vi "FXP_AFMss_MPC_singleAxis.vi"() -> ()   [LabVIEW 2017]
uses:
  <vilib>/eio/EIONode/EIONode.xnode
  <vilib>/rvi/eio/common/nirviEmuTemplateMethod_errors.vi
  <vilib>/rvi/DataTransferAndStorage/Container/XNode/niFpgaContainer.xnode
  <vilib>/eio/EIOGrowableMethodNode/genericMethod/EIOGrowableMethodNode.xnode
  <vilib>/rvi/eio/nirviErrorMerge/nirviErrorMerge.xnode
  <vilib>/rvi/eio/nirviEIOMethodImplementation/nirviEIOMethodImplementation.xnode
  <vilib>/rvi/eio/common/nirviEmuClasses.ctl
  <vilib>/rvi/FXPMathLib/FxpSub/XNode/nifxpmath_Sub.xnode
  <vilib>/Platform/TimedLoop/XDataNode/XDataNode.xnode
  <vilib>/Platform/TimedLoop/XDataNode/nitl_modes.ctl
  <vilib>/Platform/TimedLoop/XDataNode/XDNodeRunTimeDep.lvlib
  <vilib>/Platform/TimedLoop/XDataNode/wakeup.ctl
  <vilib>/Platform/TimedLoop/XDataNode/timing_clust.ctl
  <vilib>/rvi/FXPMathLib/sim/FxpSim.dll
  <vilib>/rvi/interface/RandomDataEmulation/nirviRandomDataFpgaReadWriteTemplate.vi
  fpga_fp_interface_lib/fpga_interface_types/boolean_indicators.ctl
  <vilib>/rvi/Memory/Memory_Emulation/nirvimemoryFastEmulation.vi
  <vilib>/rvi/Memory/Memory_Emulation/nirvimemoryEmulation.vi
  typeDefs/FXPControlParams_distEst.ctl
  fgm_pipiline/quadProgParams_pipe.ctl
panel:
  in  "ControlParams_distEst":T1={"umax"=3.0, "NS"=0, "ref_f_VEC"=[0.0, 0.0], "du_max"=0.0}
  in  "QP_params":T2={"maxIter"=0, "nuN"=24, "Ns_mpc"=0, "-beta"=-0.9987945556640625, "beta+1"=1.9987945556640625}
  out "Matrix FIFO \nTimeOut":bool
  out "u_k out":fxp<+/-,32,5>
  out "boolean  indicators":T3
  out "x-x(0)":fxp<+/-,18,5>
  out "y-axis fast":fxp<+/-,16,5>
  out "x(0)":fxp<+/-,16,5>
  out "LoopTicks2":u32
  out "Error Out":errorcluster
  out "x-axis fast":fxp<+/-,16,5>
  out "AI Timed Out":bool
  out "Stopped":bool
  in  "Settle Ticks":i16=1000
  in  "iters":i16=1
  in  "ymax":fxp<+/-,32,16>=4.0
  in  "TsTicks":i16
  out "Loop Ticks (benchmark)":i16
  out "NS":u8=2
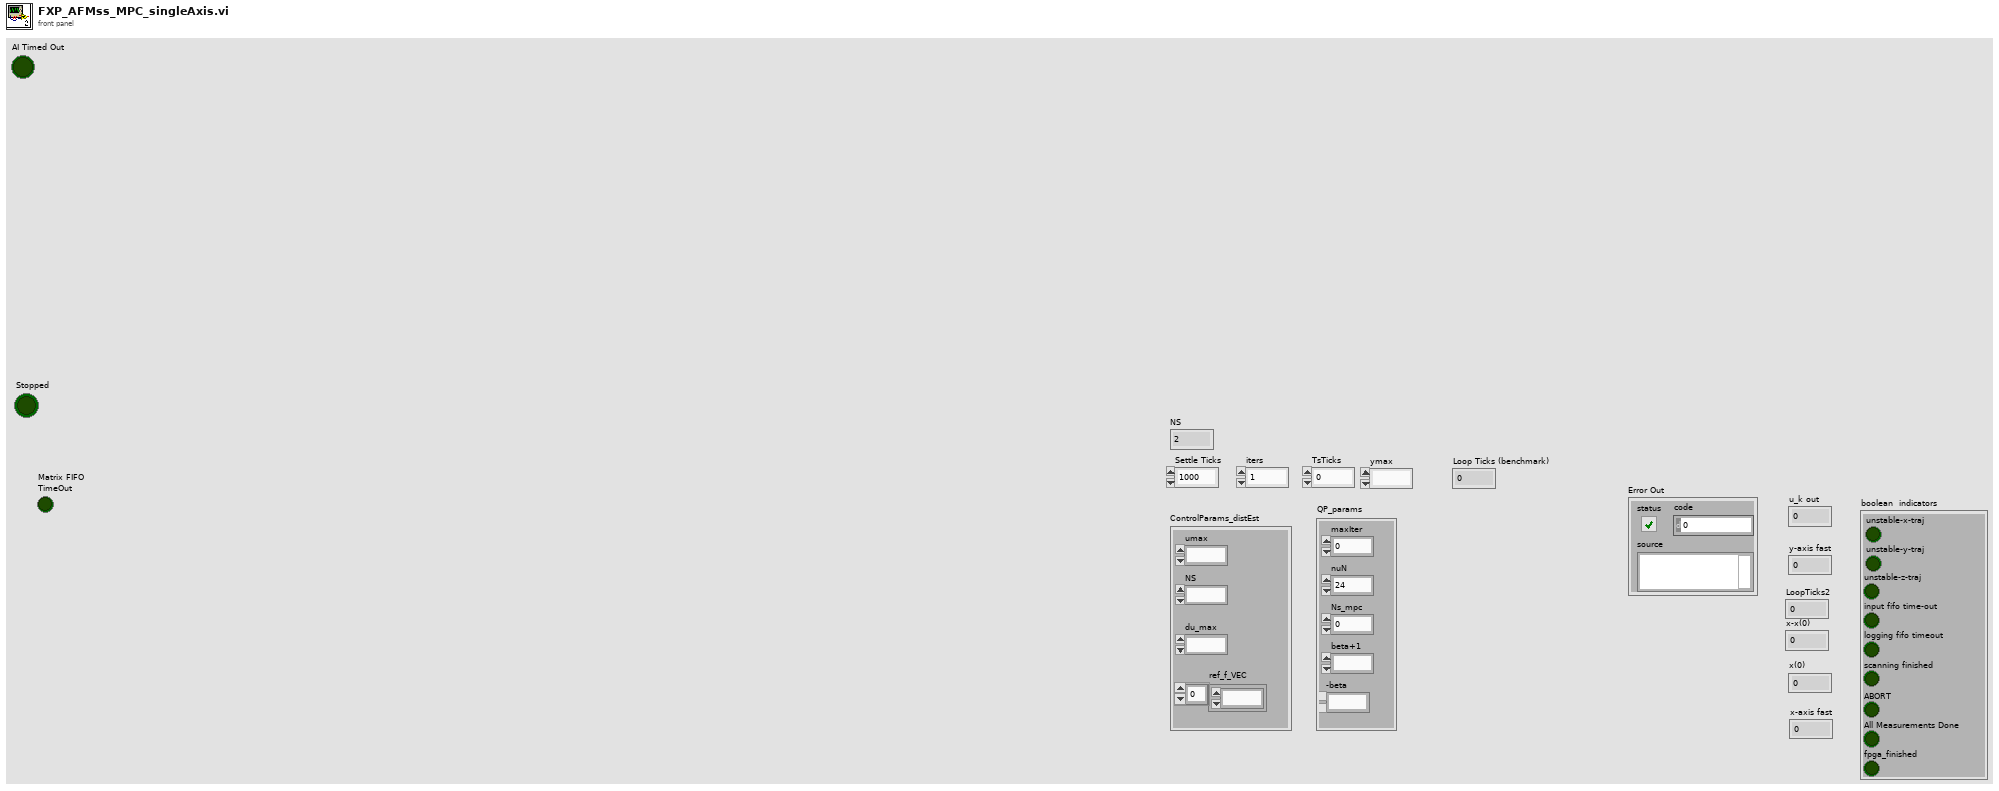
[diagram p1: front panel]
types:
  T1 = typedef "FXPControlParams_distEst.ctl" = cluster{"umax":fxp<+/-,18,5>, "NS":u8, "ref_f_VEC":fxp<+/-,32,5>[], "du_max":fxp<+/-,18,5>}
  T2 = typedef "quadProgParams_pipe.ctl" = cluster{"maxIter":u16, "nuN":u16, "Ns_mpc":u16, "-beta":fxp<+/-,18,2>, "beta+1":fxp<+/-,18,2>}
  T3 = typedef "boolean_indicators.ctl" = cluster{"unstable-z-traj":bool, "input fifo time-out":bool, "logging fifo timeout":bool, "scanning finished":bool, "unstable-x-traj":bool, "unstable-y-traj":bool, "ABORT":bool, "All Measurements Done":bool, "fpga_finished":bool}
  T4 = typedef "nirviEmuClasses.ctl" = enum16{"IO Read", "IO Write", "Method", "Property Read", "Property Write"}
  T5 = typedef "XDNodeRunTimeDep.lvlib/timing_clust.ctl" = cluster{"Expected End [f-1]":u64, "Actual End [f-1]":u64, "Finished Late? [f-1]":bool, "Expected End [i-1]":u64, "Actual End [i-1]":u64, "Finished Late? [i-1]":bool, "Expected Start [i]":u64, "Actual Start [i]":u64, "Expected Start [f]":u64, "Actual Start [f]":u64, "Source Name":string, "Structure Name":string, "Period":i64, "Deadline":i64, "Offset":i64, "Start":i64, "Priority":i32, "Timeout":i32, "Mode":T6, "Wakeup Reason":T7, "Error":errorcluster, "Source Type":string, "Secondary Source Type":string, "Global End Time":u64, "Global Start Time":u64, "Frame Duration":u64, "Iteration Duration":u64, "Assigned CPU":i32, "I/O Scan Engine Mode":u32}
  T6 = typedef "XDNodeRunTimeDep.lvlib/nitl_modes.ctl" = enum32{"No Change", "Process missed periods, maintain original phase", "Discard missed periods, maintain original phase", "Process missed periods, ignore original phase", "Discard missed periods, ignore original phase"}
  T7 = typedef "XDNodeRunTimeDep.lvlib/wakeup.ctl" = enum32{"Normal", "Aborted", "Asynchronous wakeup", "Timing source error", "Timed loop error", "Timeout"}
  T8 = typedef "x_vec_type.ctl" = fxp<+/-,32,6>[]
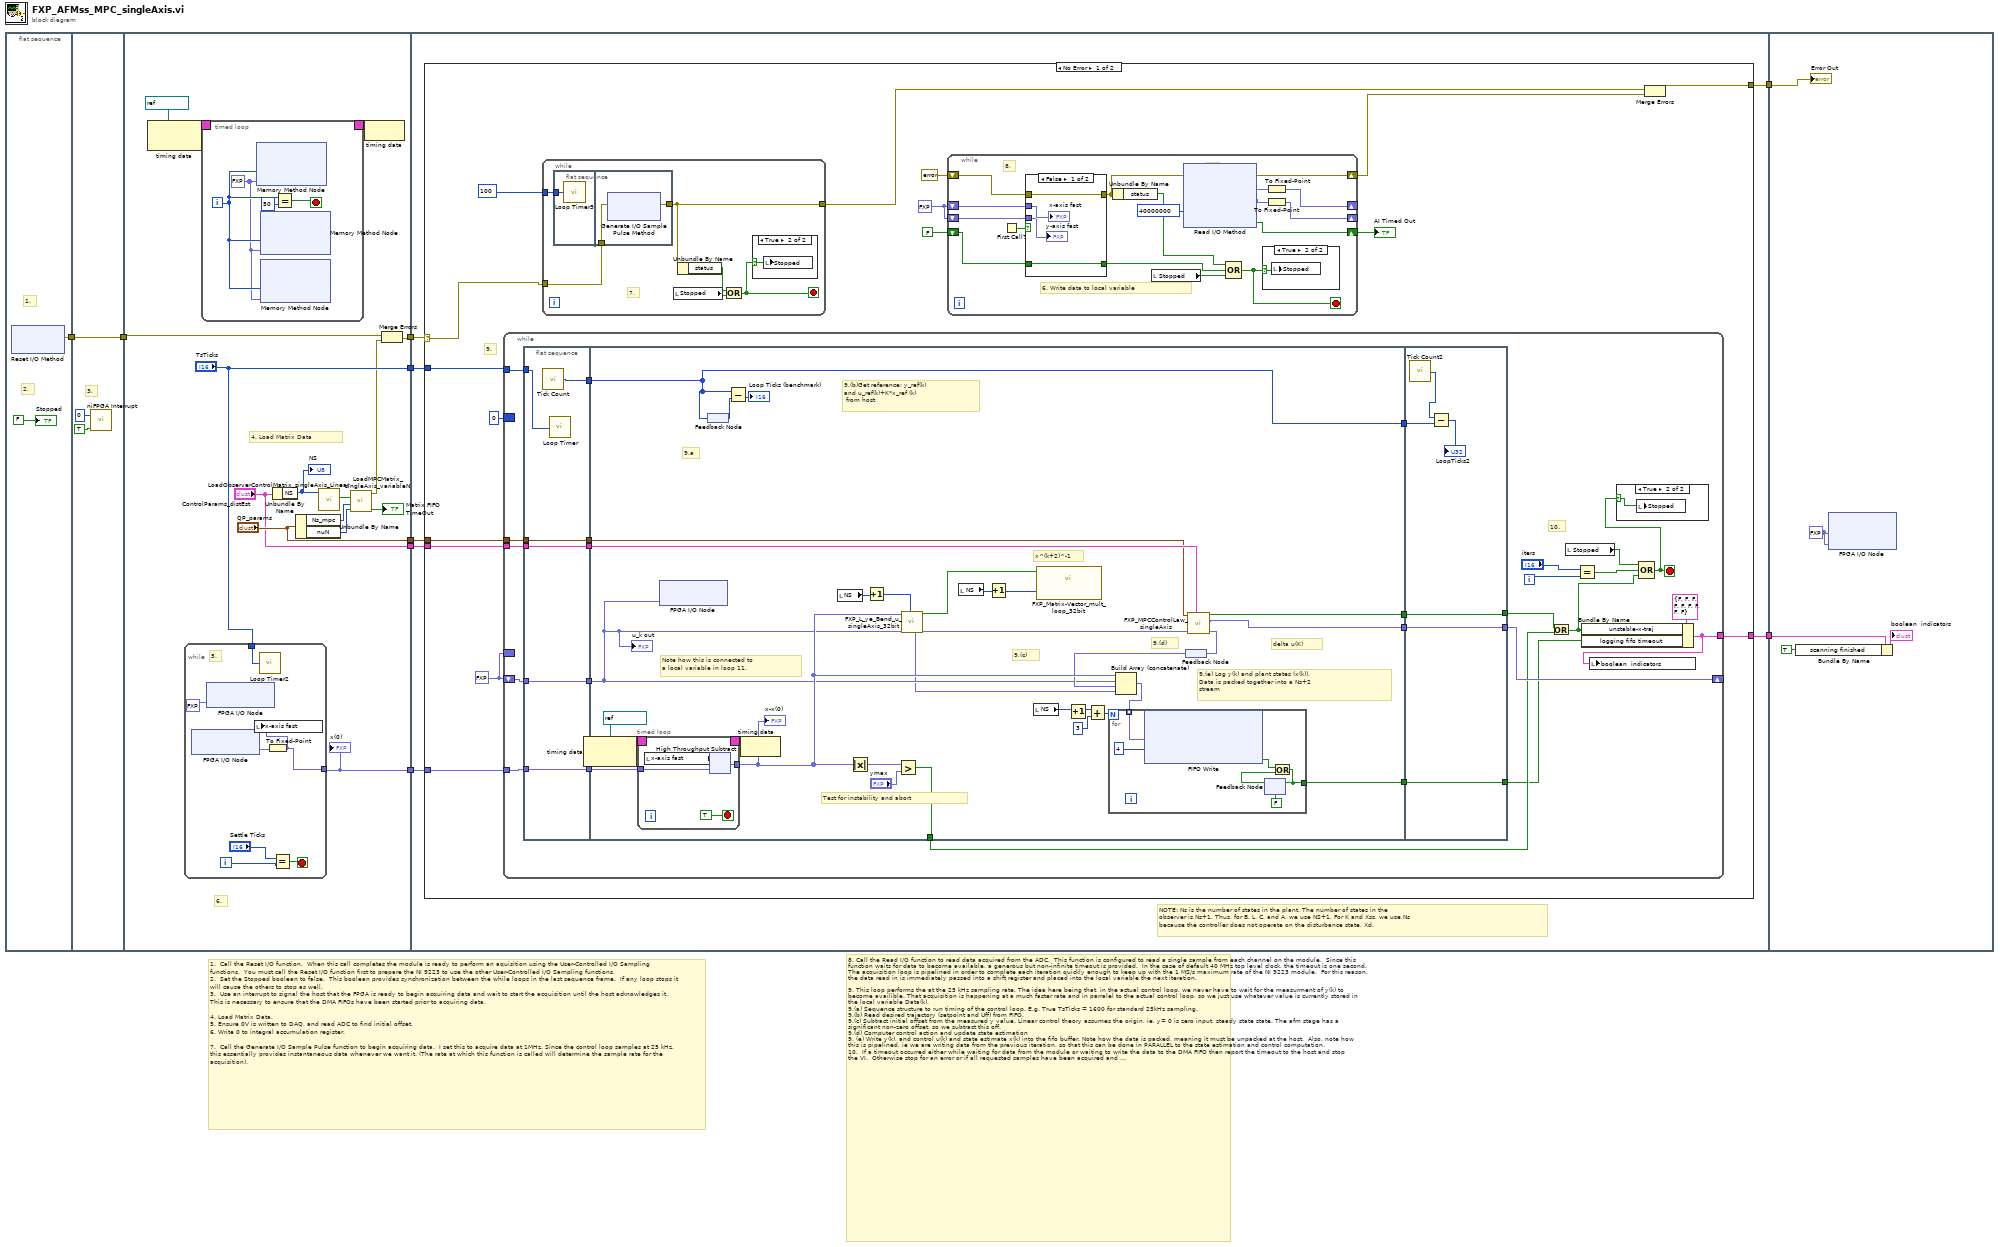
[diagram p0: block diagram]
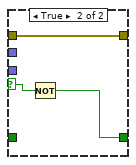
[diagram p2: hidden frame]
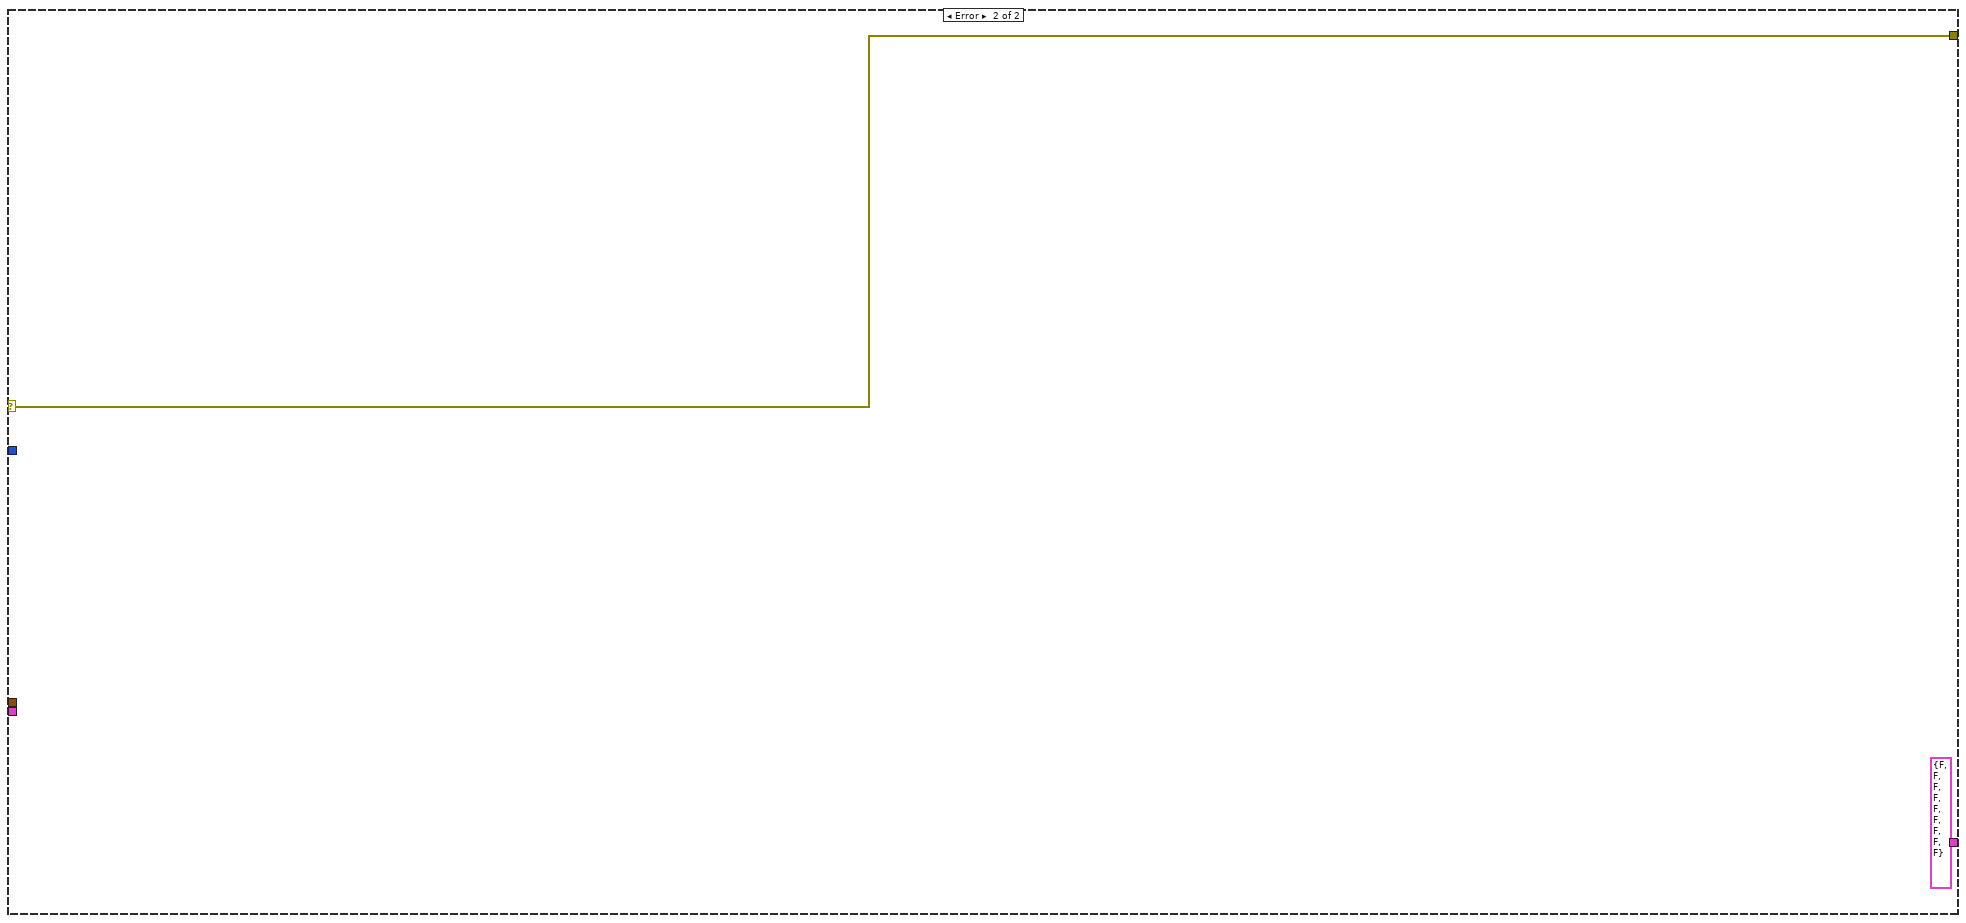
[diagram p6: hidden frame]
diagram:
  # "8. Call the Read I/O function to read data acquired from the ADC.  This function is configured to read a single sample from each channel on the module.  Since this function waits for data to become available, a generous but non-infinite timeout is provided.  In the case of default 40 MHz top level clock, the timeout is one second.  The acquisition loop is pipelined in order to complete each iteration quickly enough to keep up with the 1 MS/s maximum rate of the NI 9223 module.  For this reason, the data read in is immediately passed into a shift register and placed into the local variable the next iteration.\n\n9. This loop performs the at the 25 kHz sampling rate. The idea here being that, in the actual control loop, we never have to wait for the measurment of y(k) to become availible. That acquisition is happening at a much faster rate and in parralel to the actual control loop, so we just use whatever value is currently stored in the local variable Data(k).\n9.(a) Sequence structure to run timing of the control loop. E.g. True TsTicks = 1600 for standard 25kHz sampling.\n9.(b) Read desired trajectory (setpoint and Uff) from FIFO.\n9.(c) Subtract initial offset from the measured y value. Linear control theory assumes the origin, ie, y= 0 is zero input, steady state state. The afm stage has a significant non-zero offset, so we subtract this off.\n9.(d) Computer control action and update state estimation\n9. (e) Write y(k), and control u(k) and state estimate x(k) into the fifo buffer. Note how the data is packed, meaning it must be unpacked at the host.  Also, note how this is pipelined, ie we are writing data from the previous iteration, so that this can be done in PARALLEL to the state estimation and control computation.  \n10.  If a timeout occurred either while waiting for data from the module or waiting to write the data to the DMA FIFO then report the timeout to the host and stop the VI.  Otherwise stop for an error or if all requested samples have been acquired and placed into the DMA FIFO or if the controll law has detected instability.\n\n11. WRITE  TO DAQ. Note how the output of the control law is connected to loop 11 through a local variable."
  # "1.  Call the Reset I/O function.  When this call completes the module is ready to perform an aquisition using the User-Controlled I/O Sampling functions.  You must call the Reset I/O function first to prepare the NI 9223 to use the other User-Controlled I/O Sampling functions.\n2.  Set the Stopped boolean to false.  This boolean provides synchronization between the while loops in the last sequence frame.  If any loop stops it will cause the others to stop as well.\n3.  Use an interrupt to signal the host that the FPGA is ready to begin acquiring data and wait to start the acquisition until the host acknowledges it.  This is necessary to ensure that the DMA FIFOs have been started prior to acquiring data.\n\n4. Load Matrix Data.\n5. Ensure 0V is written to DAQ, and read ADC to find initial offset.\n6. Write 0 to integral accumulation register.\n\n7.  Call the Generate I/O Sample Pulse function to begin acquiring data.  I set this to acquire data at 1MHz. Since the control loop samples at 25 kHz, this essentially provides instantaneous data whenever we want it. (The rate at which this function is called will determine the sample rate for the acquisition)."
  n1 = flat-sequence {
    tunnel: [w10] -> w4
    tunnel: [w56] -> w5
    tunnel: w4 -> [w56]
    tunnel: ["TsTicks"] -> w9
    tunnel: [w73] -> w8
    tunnel: ["ControlParams_distEst"] -> w7
    tunnel: [w62] -> w6
    tunnel: w5 -> [w61]
    tunnel: ["QP_params"] -> w1
    tunnel: w9 -> [w97]
    tunnel: w8 -> [w96]
    tunnel: w7 -> [w95]
    tunnel: w6 -> [w94]
    tunnel: [w93] -> w3
    tunnel: [w92] -> w2
    tunnel: w1 -> [w91]
    tunnel: w3 -> [w393]
    tunnel: w2 -> [w391]
    frame #0 {
      # "2."
      # "1."
      n2 = xnode "Reset I/O Method"() -> ("error out"=w10:errorcluster)  [unwired: 2 in, 1 out]
      "Stopped" <- FALSE ("Stopped")
    }
    frame #1 {
      # "3."
      n3 = call <vilib>:"niFPGA Interrupt.vi"("Wait Until Cleared (F)"=TRUE, "IRQ Number (0)"=u8 0) -> ()  [unwired: 1 in]
    }
    frame #2 {
      # "6."
      # "4. Load Matrix Data"
      n4 = node-c288(refnum<k21> "80MHz" ("Source Name")) -> (w71:T5)
      n5 = while {
        tunnel: [w88] -> w73
        tunnel: "TsTicks" -> [w90]
        i -> [w84]
        stop <- w86 stop-if-true
        # "5."
        n6 = xnode "FPGA I/O Node"() -> ("Mod2/AI0"=w89:fxp<+/-,24,5>)  [unwired: 1 in, 1 out]
        n7 = xnode "FPGA I/O Node"("Mod1/AO0"=fxp<+,1,1> 0.0) -> ()  [unwired: 1 in, 1 out]
        n8 = call "Loop Timer2"("Count(Ticks)"=w90) -> ()  [unwired: 1 out]
        n9 = To Fixed-Point(number=w89) -> (fixed-point=w88:fxp<+/-,16,5>)  [unwired: 1 in]
        n10 = local write "x-axis fast"(w88) -> ()
        n11 = Equal?(x="Settle Ticks", y=w84) -> (x = y?=w86:bool)
      }
      "x(0)" <- w73
      n12 = timed-loop {
        timing: w71 -> [_]
        timing-out: [_] -> w70
        i -> [w75]
        stop <- w77 stop-if-true
        w74 = fxp<+/-,32,5> 0.0 ("Data")
        n13 = xnode ("Memory Method Node")("Address"=w75, "Data"=w74) -> ()  [unwired: 1 in, 1 out]
        n14 = xnode ("Memory Method Node")("Address"=w75, "Data"=w74) -> ()  [unwired: 1 in, 1 out]
        n15 = xnode ("Memory Method Node")("Address"=w75, "Data"=w74) -> ()  [unwired: 1 in, 1 out]
        n16 = Equal?(x=w75, y=50) -> (x = y?=w77:bool)
      }
      n17 = Unbundle By Name("ControlParams_distEst") -> ("NS"=w68:u8)
      "NS" <- w68
      n18 = Unbundle By Name("QP_params") -> ("Ns_mpc"=w65:u16, "nuN"=w64:u16)
      n19 = call "LoadObserverControlMatrix_singleAxis_Linear.vi"("NS"=w68) -> ("SS FIFO TimeOut?"=w66:bool)  [unwired: 10 in]
      n20 = call "LoadMPCMatrix_singleAxis_variableN.vi"("nuN_mpc"=w64, "Ns+1"=w65, "FIFO Timeout\nIn"=w66) -> ("FIFO Matrix Timeout"=→"Matrix FIFO \nTimeOut":bool, "error out"=w63:errorcluster)  [unwired: 7 in]
      n21 = node-c288(w70) -> ()
      n22 = Merge Errors(w61, w63) -> (w62:errorcluster)
    }
    frame #3 {
      # "NOTE: Ns is the number of states in the plant. The number of states in the \nobserver is Ns+1. Thus, for B, L, C, and A, we use NS+1. For K and Xss, we use Ns\nbecause the controller does not operate on the disturbance state, Xd."
      n23 = case shown="No Error" w94 {
        selector: w94 -> [w102 w388]
        tunnel: w97 -> [w104 _]
        tunnel: w96 -> [w105 _]
        tunnel: w95 -> [w112 _]
        tunnel: [w109 w388] -> w93
        tunnel: [w100 T3 {"unstable-z-traj"=FALSE, "input fifo time-out"=FALSE, "logging fifo timeout"=FALSE, "scanning finished"=FALSE, "unstable-x-traj"=FALSE, "unstable-y-traj"=FALSE, "ABORT"=FALSE, "All Measurements Done"=FALSE, "fpga_finished"=FALSE} ("boolean  indicators 2")] -> w92
        tunnel: w91 -> [w98 _]
        frame No Error {
          w101 = fxp<+/-,18,5> 0.0
          w103 = fxp<+/-,16,5> 0.0 ("Mod1/AI0")
          # "9."
          n24 = while {
            border: i16 0 -> [_]
            tunnel: w112 -> [w324]
            shift-right: [w312] -> _
            shift-left: w101 -> [w322]
            tunnel: w105 -> [w321]
            tunnel: w104 -> [w313]
            border: w101 -> [_]
            tunnel: [w307] -> w100
            tunnel: w98 -> [w301]
            i -> [w325]
            stop <- w304 stop-if-true
            # "10."
            n25 = flat-sequence {
              tunnel: w321 -> [w331]
              tunnel: w322 -> [w332]
              tunnel: w324 -> [w333]
              tunnel: [w333] -> w317
              tunnel: [w332] -> w316
              tunnel: [w331] -> w315
              tunnel: [w330] -> w314
              tunnel: w313 -> [w329]
              tunnel: [w328] -> w302
              tunnel: w301 -> [w328]
              tunnel: [w363] -> w308
              tunnel: [w337] -> w320
              tunnel: [w364] -> w319
              tunnel: [w362] -> w318
              tunnel: w314 -> [w362]
              tunnel: w315 -> [w353]
              tunnel: w316 -> [w346]
              tunnel: w317 -> [w339]
              tunnel: [w338] -> w311
              tunnel: w302 -> [w334]
              tunnel: [w386] -> w303
              tunnel: w320 -> [w382]
              tunnel: w319 -> [w386]
              tunnel: w318 -> [w384]
              tunnel: [w382] -> w312
              tunnel: [w381] -> w309
              tunnel: w311 -> [w381]
              frame #0 {
                n26 = call "Tick Count"() -> ("Tick Count(Ticks)"=w330:u32)
                n27 = call "Loop Timer"("Count(Ticks)"=w329) -> ()  [unwired: 1 out]
              }
              frame #1 {
                # "delta u(K)"
                # "Note how this is connected to\na local variable in loop 11."
                # "9.a"
                # "x^(k+2)^-1"
                # "9.(c)"
                # "9.(b)Get reference: y_ref(k)\nand u_ref(k)+K*x_ref (k)\n from host"
                # "9.(d)"
                # "9.(e) Log y(k) and plant states (x(k)). \nData is packed together into a Ns+2 \nstream"
                # "Test for instability and abort"
                n28 = node-c288(refnum<k21> "80MHz" ("Source Name")) -> (w357:T5)
                n29 = timed-loop {
                  timing: w357 -> [_]
                  timing-out: [_] -> w356
                  tunnel: w353 -> [w367]
                  tunnel: [w366] -> w348
                  stop <- TRUE stop-if-true
                  n30 = local read "x-axis fast"() -> (w368:fxp<+/-,16,5>)
                  n31 = xnode "High Throughput Subtract"("x"=w368, "y"=w367) -> ("x-y"=w366:fxp<+/-,18,5>)
                }
                "x-x(0)" <- w348
                n32 = xnode "FPGA I/O Node"("Mod1/AO0"=w346) -> ()  [unwired: 1 in, 1 out]
                n33 = feedback #1() -> (w354:u32)
                n34 = feedback-in #1(w362) -> ()
                n35 = Subtract(x=w362, y=w354) -> (x-y=→"Loop Ticks (benchmark)":u32)
                n36 = node-c288(w356) -> ()
                n37 = local read "NS"() -> (w358:u8)
                n38 = Absolute Value(x=w348) -> (abs(x)=w361:fxp<+,18,5>)
                n39 = Increment(x=w358) -> (x+1=w350:u8)
                n40 = Greater?(x=w361, y="ymax") -> (0:w363:bool)
                n41 = call "FXP_L_ye_Bend_u_singleAxis_32bit.vi"("NS"=w350, "U(k): ux"=w346, "Y(k): x"=w348) -> ("yd_est"=w335:fxp<+/-,32,5>, "outputValid"=w351:bool, "x0"=w340:T8)  [unwired: 6 in]
                n42 = local read "NS"() -> (w359:u8)
                n43 = Increment(x=w359) -> (x+1=w349:u8)
                n44 = local read "NS"() -> (w344:u8)
                n45 = call "FXP_Matrix-Vector_mult_loop_32bit.vi"("Ns_2"=w349, "inputValid"=w351) -> ()  [unwired: 9 in, 1 out]
                n46 = Increment(x=w344) -> (x+1=w343:u8)
                n47 = Add(x=w343, y=u8 3) -> (x+y=w341:u8)
                n48 = feedback #2() -> (w347:fxp<+/-,64,15>)
                n49 = Build Array (concatenate)(w348, w346, w347, w340) -> (w345:fxp<+/-,64,15>[])
                n50 = for {
                  N: w341 -> [_]
                  tunnel: w345 -> [w379] mode=indexing
                  tunnel: [w375] -> w364
                  n51 = xnode ("FIFO Write")("Element"=w379, "Timeout"=i16 4) -> ("Timed Out?"=w378:bool)  [unwired: 1 in, 1 out]
                  n52 = feedback #3(FALSE) -> (w377:bool)
                  n53 = Or(x=w378, y=w377) -> (x .or. y?=w375:bool)
                  n54 = feedback-in #3(w375) -> ()
                }
                n55 = call "FXP_MPCControlLaw_singleAxis.vi"("ControlParams_distEst"=w339, "yd_est_x"=w335, "QP_params"=w334) -> ("del u_x"=w336:fxp<+/-,64,15>, "u_k (saturated)"=w337:fxp<+/-,32,5>, "saturated?"=w338:bool)  [unwired: 6 in]
                n56 = feedback-in #2(w336) -> ()
                "u_k out" <- w346
              }
              frame #2 {
                n57 = call "Tick Count2"() -> ("Tick Count(Ticks)"=w385:u32)
                n58 = Subtract(x=w385, y=w384) -> (x-y=→"LoopTicks2":u32)
              }
            }
            n59 = Or(x=w309, y=w308) -> (x .or. y?=w305:bool)
            n60 = local read "Stopped"() -> (w306:bool)
            n61 = Equal?(x="iters", y=w325) -> (x = y?=w323:bool)
            n62 = Bundle By Name(cluster=T3 {"unstable-z-traj"=FALSE, "input fifo time-out"=FALSE, "logging fifo timeout"=FALSE, "scanning finished"=FALSE, "unstable-x-traj"=FALSE, "unstable-y-traj"=FALSE, "ABORT"=FALSE, "All Measurements Done"=FALSE, "fpga_finished"=FALSE} ("boolean  indicators"), "unstable-x-traj"=w305, "logging fifo timeout"=w303) -> (w307:T3)
            n63 = local write "boolean  indicators"(w307) -> ()
            n64 = Compound Arithmetic op=OR(w306, w323, w305) -> (w304:bool)
            n65 = case shown="True" w304 {
              selector: w304 -> [_ w327]
              frame False {
              }
              frame True {
                n66 = local write "Stopped"(w327) -> ()
              }
            }
          }
          n67 = while {
            tunnel: u32 100 ("Max TsTicks") -> [w252]
            tunnel: [w249] -> w107
            tunnel: w102 -> [w247]
            stop <- w248 stop-if-true
            # "7."
            n68 = flat-sequence {
              tunnel: w252 -> [w254]
              tunnel: [w256] -> w249
              tunnel: w247 -> [w255]
              frame #0 {
                n69 = call "Loop Timer3"("Count(Ticks)"=w254) -> ()  [unwired: 1 out]
              }
              frame #1 {
                n70 = xnode "Generate I/O Sample Pulse Method"("error in"=w255) -> ("error out"=w256:errorcluster)  [unwired: 1 in, 1 out]
              }
            }
            n71 = local read "Stopped"() -> (w251:bool)
            n72 = Unbundle By Name(w249) -> ("status"=w250:bool)
            n73 = Compound Arithmetic op=OR(w250, w251) -> (w248:bool)
            n74 = case shown="True" w248 {
              selector: w248 -> [_ w253]
              frame False {
              }
              frame True {
                n75 = local write "Stopped"(w253) -> ()
              }
            }
          }
          n76 = while {
            shift-right: [w129] -> w106
            shift-left: errorcluster {"status"=FALSE, "code"=0, "source"=""} ("error out") -> [w123]
            shift-right: [w128] -> w108
            shift-left: FALSE ("Timed Out") -> [w120]
            shift-right: [w118] -> _
            shift-left: w103 -> [w124]
            shift-right: [w116] -> _
            shift-left: w103 -> [w115]
            stop <- w127 stop-if-true
            # "8."
            # "6. Write data to local variable"
            # "5."
            n77 = First Call?() -> (First Call?: T/F=w121:bool)
            n78 = case shown="False" w121 {
              selector: w121 -> [_ w136]
              tunnel: [w132 w135] -> w125
              tunnel: w124 -> [w133 _]
              tunnel: w123 -> [w134 w137]
              tunnel: [w134 w137] -> w114
              tunnel: w120 -> [w132 _]
              tunnel: w115 -> [w131 _]
              frame False {
                "x-axis fast" <- w133
                "y-axis fast" <- w131
              }
              frame True {
                n79 = Not(x=w136) -> (.not. x?=w135:bool)
              }
            }
            n80 = Unbundle By Name(w114) -> ("status"=w122:bool)
            n81 = local read "Stopped"() -> (w126:bool)
            n82 = xnode "Read I/O Method"("error in"=w114, "Timeout"=40000000) -> ("error out"=w129:errorcluster, "Mod2/AI0"=w119:fxp<+/-,24,5>, "Mod2/AI1"=w117:fxp<+/-,24,5>, "Timed Out"=w128:bool)  [unwired: 2 in, 2 out]
            n83 = Compound Arithmetic op=OR(w122, w125, w126) -> (w127:bool)
            n84 = case shown="True" w127 {
              selector: w127 -> [_ w138]
              frame False {
              }
              frame True {
                n85 = local write "Stopped"(w138) -> ()
              }
            }
            n86 = To Fixed-Point(number=w119) -> (fixed-point=w118:fxp<+/-,16,5>)  [unwired: 1 in]
            n87 = To Fixed-Point(number=w117) -> (fixed-point=w116:fxp<+/-,16,5>)  [unwired: 1 in]
          }
          "AI Timed Out" <- w108
          n88 = Merge Errors(w107, w106) -> (w109:errorcluster)
        }
        frame Error {
        }
      }
    }
    frame #4 {
      w392 = fxp<+/-,20,5> 0.0 ("Mod1/AO0")
      n89 = Bundle By Name(cluster=w391, "scanning finished"=TRUE) -> (→"boolean  indicators":T3)
      n90 = xnode "FPGA I/O Node"("Mod1/AO0"=w392, "Mod1/AO1"=w392) -> ()  [unwired: 2 in, 2 out]
      "Error Out" <- w393
    }
  }
